vi "SVPO RMS Level (1 Ch DBL WDT) with IC.vi"(6 "restart averaging? (F)":bool, 8 "initial conditions":T1, 11 "scaled signal [EU]":waveform(dbl)={"t0"=timestamp(0 s since 1904-01-01), "dt"=0.0, "Y"=[]}) -> (0 "final conditions":T1, 3 "RMS level":dbl=nan, 4 "duration [s]":dbl, 5 "timestamp":timestamp)   [LabVIEW 2017, in "SoundVib_VibrationLevel.lvlib"]
doc: "Computes the root-mean-square (RMS) level of scaled time waveform signals and scaled array signals. <B>scaled signal [EU]</B> should have a zero DC component. You can attenuate the DC component with hardware AC-coupling filters and with software high-pass filters. Use this VI on embedded targets that have limited computational resources. Wire data to the <B>scaled signal [EU]</B> input to determine the polymorphic instance to use or manually select the instance."
uses:
  <vilib>/addons/Sound and Vibration/svt_Level/SoundVib_VibrationLevel.lvlib
  <vilib>/addons/_NISVFA/_Shared subVIs/Controls/svc_RMS Level State.ctl
  <vilib>/Analysis/baseanly.llb/Dot Product.vi
  <vilib>/Analysis/baseanly.llb/Real Dot Product.vi
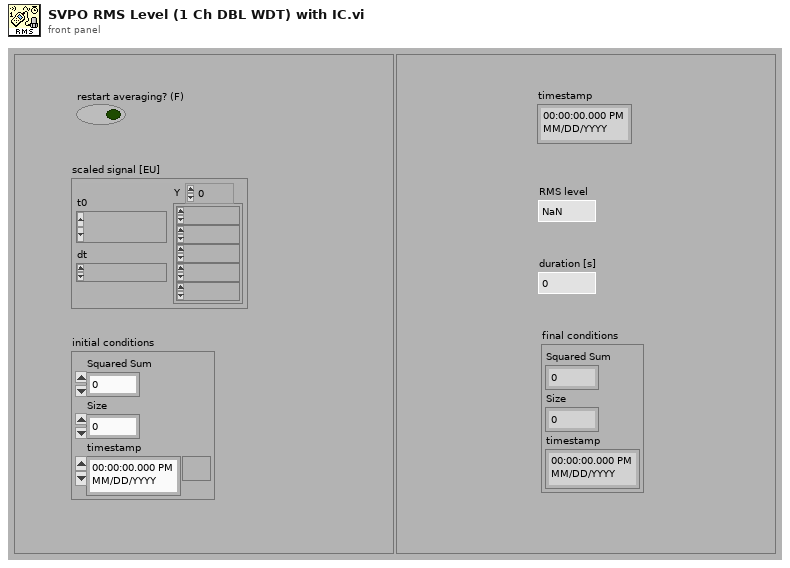
[diagram p1: front panel]
types:
  T1 = typedef "svc_RMS Level State.ctl" = cluster{"Squared Sum":dbl, "Size":u64, "timestamp":timestamp}
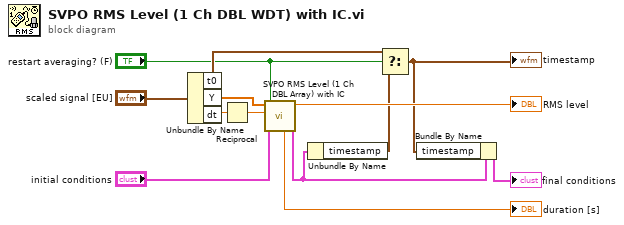
[diagram p0: block diagram]
diagram:
  n1 = Unbundle By Name("scaled signal [EU]") -> ("t0"=w11:timestamp, "Y"=w8:dbl[], "dt"=w10:dbl)
  n2 = Reciprocal(x=w10) -> (1/x=w9:dbl)
  n3 = call <vilib>:"SVPO RMS Level (1 Ch DBL Array) with IC.vi"("restart averaging? (F)"="restart averaging? (F)", "initial conditions"="initial conditions", "sampling rate [Hz]"=w9, "scaled signal [EU]"=w8) -> ("final conditions"=w1:T1, "RMS level"=→"RMS level":dbl, "duration [s]"=→"duration [s]":dbl)  [unwired: 5 in]
  n4 = Unbundle By Name(w1) -> ("timestamp"=w4:timestamp)
  n5 = Select(t=w11, s="restart averaging? (F)", f=w4) -> (s? t:f=w3:timestamp)
  "timestamp" <- w3
  n6 = Bundle By Name(cluster=w1, "timestamp"=w3) -> (→"final conditions":T1)
